vi "Status Read stop.vi"(8 "error in (no error)":errorcluster, 11 "Status Reference":T1) -> (0 "error out":errorcluster, 1 "Stop":bool, 3 "Status Reference out":T1)   [LabVIEW 2019, in "Status.lvlib"]
uses:
  Status.lvlib
  Ctl/control.ctl
  Ctl/State.ctl
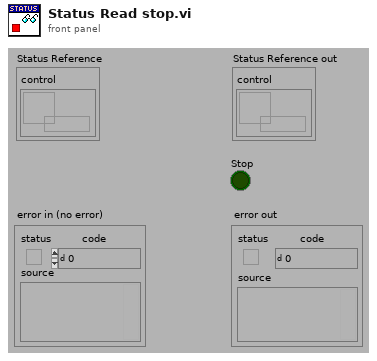
[diagram p1: front panel]
types:
  T1 = typedef "Status.lvlib/control.ctl" = cluster{"control":refnum<data-value>}
  T2 = typedef "Status.lvlib/State.ctl" = enum8{"initialization", "redefine", "standby", "connect", "wait to reconnect", "wait to reset timeout", "configure", "requests", "close connection", "stop"}
  T3 = cluster{"set_state":cluster{"Start":bool, "WrEn":bool, "Stop":bool}, "state":cluster{"errors":i32, "connect":bool, "state":T2}}
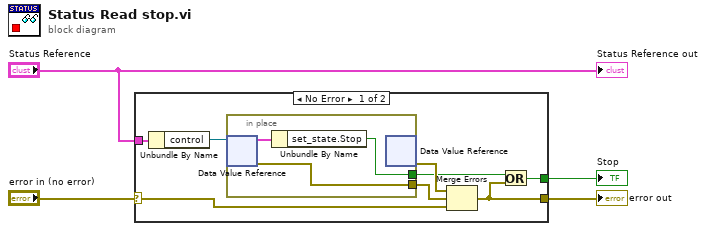
[diagram p0: block diagram]
diagram:
  n1 = case shown="No Error" "error in (no error)" {
    selector: "error in (no error)" -> [w8 w16]
    tunnel: [w7 w16] -> w3
    tunnel: [w6 _] -> w2
    tunnel: "Status Reference" -> [w12 _]
    frame No Error {
      n2 = Unbundle By Name(w12) -> ("control"=w10:refnum<data-value>)
      n3 = in-place {
        in-place-border: [w15] -> w9
        in-place-border: [w13] -> w5
        n4 = in-place-dvr #1(w10) -> (w14:T3, w15:errorcluster)
        n5 = Unbundle By Name(w14) -> ("set_state.Stop"=w13:bool)
        n6 = in-place-dvr #1() -> (w11:errorcluster)  [unwired: 1 in, 1 out]
      }
      n7 = Merge Errors(w11, w9, w8) -> (w7:errorcluster)
      n8 = Or(x=w5, y=w7) -> (x .or. y?=w6:bool)
    }
    frame Error {
    }
  }
  "error out" <- w3
  "Stop" <- w2
  "Status Reference out" <- "Status Reference"
